vi "niFPGA U64xU16 - MSB.vi"(2 "A":u64, 3 "B":u16) -> (7 "A*B [Hi I64]":u64=2838 format="%08x")   [LabVIEW 2017]
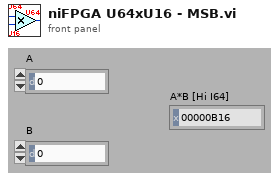
[diagram p1: front panel]
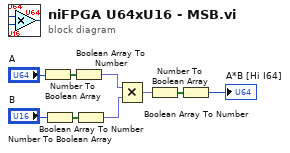
[diagram p0: block diagram]
diagram:
  n1 = Number To Boolean Array(number="A") -> (Boolean array=w8:bool[])
  n2 = Number To Boolean Array(number="B") -> (Boolean array=w9:bool[])
  n3 = Boolean Array To Number(Boolean array=w8) -> (number=w7:fxp<+,64,0>)
  n4 = Boolean Array To Number(Boolean array=w9) -> (number=w6:fxp<+,16,0>)
  n5 = Multiply(x=w7, y=w6) -> (x*y=w4:fxp<+,64,0>)
  n6 = Number To Boolean Array(number=w4) -> (Boolean array=w5:bool[])
  n7 = Boolean Array To Number(Boolean array=w5) -> (number=→"A*B [Hi I64]":u64)
